vi "DestroyLVINILocalHostKey.vi"   [LabVIEW 2021]
uses:
  <vilib>/Wiresmith Technology/G CLI/CLI Class/CLI.lvclass
  <vilib>/Utility/config.llb/NI_LVConfig.lvlib
types:
  T1 = enum32{"Invalid", "Standard", "Closed", "Hidden", "Minimized", "Maximized"}
  T2 = typedef "NI_LVConfig.lvlib/Config Data RefNum.ctl" = refnum<k1>
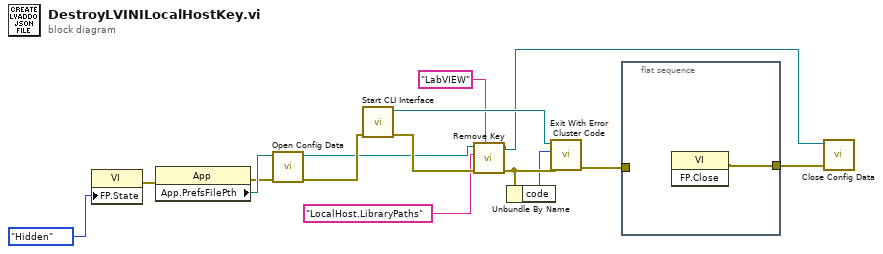
[diagram p0: block diagram]
diagram:
  n1 = property class="VI"("FP.State"=T1."Hidden" ("Front Panel Window:State")) -> (error out=w10:errorcluster)  [unwired: 2 in, 1 out]
  n2 = property class="App"(error in=w10) -> (error out=w11:errorcluster, "App.PrefsFilePth"=w12:path)  [unwired: 1 in, 1 out]
  n3 = call <vilib>:"Open Config Data.vi"("error in (no error)"=w11, "configuration file path"=w12) -> ("error out"=w9:errorcluster, "refnum"=w5:T2)  [unwired: 7 in, 1 out]
  n4 = call <vilib>:"Start CLI Interface.vi"("error in (no error)"=w9) -> ("error out"=w6:errorcluster, "CLI out"=w13:refnum<class "CLI.lvclass">)  [unwired: 7 in, 2 out]
  n5 = call <vilib>:"Remove Key.vi"("section"="LabVIEW", "error in (no error)"=w6, "key"="LocalHost.LibraryPaths", "refnum"=w5) -> ("error out"=w2:errorcluster, "refnum out"=w4:T2)  [unwired: 5 in, 1 out]
  n6 = Unbundle By Name(w2) -> ("code"=w1:i32)
  n7 = call <vilib>:"Exit With Error Cluster Code.vi"("error in (no error)"=w2, "No Error Code (0)"=w1, "CLI in"=w13) -> ("error out"=w14:errorcluster)  [unwired: 8 in]
  n8 = flat-sequence {
    tunnel: [w16] -> w8
    tunnel: w14 -> [_]
    frame #0 {
      n9 = invoke class="VI" method="FP.Close"() -> (error out=w16:errorcluster)  [unwired: 3 in, 2 out]
    }
  }
  n10 = call <vilib>:"Close Config Data.vi"("error in (no error)"=w8, "refnum"=w4) -> ()  [unwired: 8 in, 2 out]
